vi "InitUSB4000_v2.vi"(2 "error in (no error)":errorcluster, 3 "Int Time (usec)":i32=1000000, 4 "USB4000 In":T1) -> (0 "error out":errorcluster, 1 "USB4000 Out":T1)   [LabVIEW 2012]
uses:
  Controls/USB4000_Data.ctl
panel:
  out "Spect*":u32
  out "Number of Spectrometers":i32
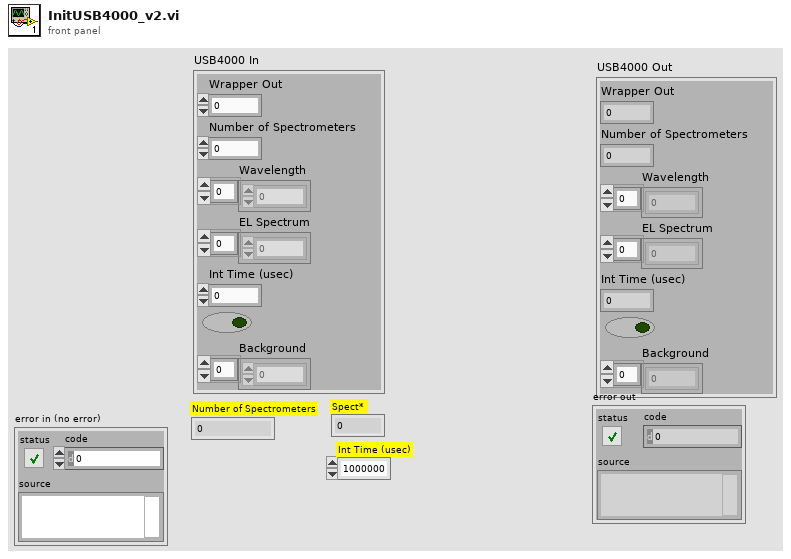
[diagram p1: front panel]
types:
  T1 = typedef "USB4000_Data.ctl" = cluster{"Wrapper Out":u32, "Number of Spectrometers":i32, "Wavelength":dbl[], "EL Spectrum":dbl[], "Int Time (usec)":i32, bool, "Background":dbl[]}
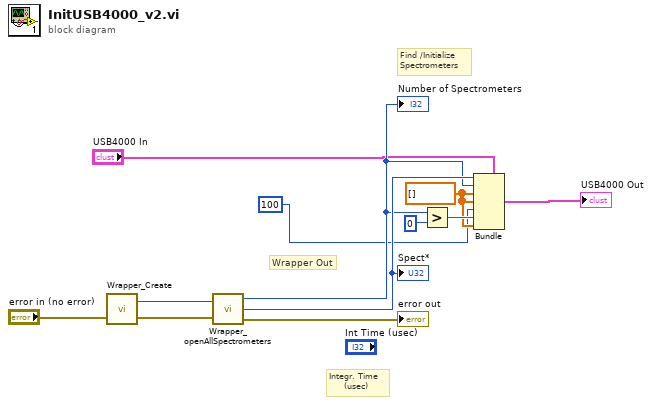
[diagram p0: block diagram]
diagram:
  w5 = dbl[] [] ("Wavelength")
  # "Integr. Time\n     (usec)"
  # "Wrapper Out"
  # "Find /Initialize\nSpectrometers"
  n1 = call "Wrapper_Create.vi"("error in (no error)"="error in (no error)") -> ("error out"=w3:errorcluster, "Wrapper"=w12:u32)  [unwired: 1 in]
  n2 = call "Wrapper_openAllSpectrometers.vi"("Wrapper In"=w12, "error in (no error)"=w3) -> ("Number of Spectrometers"=w9:i32, "Wrapper Out"=w10:u32, "error out"=→"error out":errorcluster)
  "Number of Spectrometers" <- w9
  "Spect*" <- w10
  n3 = Greater?(x=w9, y=0) -> (0:w8:bool)
  n4 = Bundle(cluster="USB4000 In", "Wrapper Out"=w10, "Number of Spectrometers"=w9, "Wavelength"=w5, "EL Spectrum"=w5, "Int Time (usec)"=100, w8, "Background"=w5) -> (→"USB4000 Out":T1)
